vi "Autonomous Independent.vi"() -> ()   [LabVIEW 2016]
doc: "This VI is called when autonomous begins, and will automatically be terminated when autonomous ends. You can carry out timed or sensor driven robot movement independently without needing to return to the caller."
uses:
  2_8_17/Auto_Action.ctl
  <vilib>/Rock Robotics/WPI/Solenoid/WPI_SolenoidValue.ctl
  <vilib>/Rock Robotics/Network Tables/NT Read Number.vi
  <vilib>/Rock Robotics/WPI/Ultrasonic/WPI_SonarSRF04DigitalRefNum Registry Get.vi
  <vilib>/Rock Robotics/WPI/Ultrasonic/WPI_SonarSRF04DigitalGetRange.vi
  FRC SimulatedRSC/Positions.vi
panel:
  in  "Value":T1=enum."Forward"
  out "Auto Mode":dbl=3.0
  in  "Auton_Modes":T3(array[cluster])=[{"Actions"=[{"Effort"=0.55, "Duration"=3.5, "Action"=enum."Nothing"}, {"Effort"=0.0, "Duration"=0.0, "Action"=enum."Nothing"}]}, {"Actions"=[{"Effort"=0.0, "Duration"=1.0, "Action"=enum."Nothing"}, {"Effort"=0.75, "Duration"=5.0, "Action"=enum."Nothing"}, {"Effort"=0.0, "Duration"=1.0, "Action"=enum."Nothing"}]}, {"Actions"=[{"Effort"=1.0, "Duration"=3.0, "Action"=enum."Nothing"}, {"Effort"=0.0, "Duration"=1.0, "Action"=enum."Nothing"}, {"Effort"=0.75, "Duration"=3.5, "Action"=enum."Nothing"}, {"Effort"=0.0, "Duration"=1.0, "Action"=enum."Nothing"}]}, {"Actions"=[{"Effort"=0.0, "Duration"=0.5, "Action"=enum."Nothing"}, {"Effort"=0.8, "Duration"=5.28, "Action"=enum."Nothing"}, {"Effort"=0.0, "Duration"=1.0, "Action"=enum."Nothing"}, {"Effort"=-0.8, "Duration"=1.8, "Action"=enum."Nothing"}, {"Effort"=0.0, "Duration"=0.1, "Action"=enum."Nothing"}, {"Effort"=0.8, "Duration"=1.75, "Action"=enum."Nothing"}, {"Effort"=0.0, "Duration"=0.5, "Action"=enum."Nothing"}, {"Effort"=0.0, "Duration"=4.0, "Action"=enum."Nothing"}]}, {"Actions"=[{"Effort"=0.0, "Duration"=0.0, "Action"=enum."Nothing"}, {"Effort"=1.0, "Duration"=0.1, "Action"=enum."Nothing"}, {"Effort"=0.0, "Duration"=0.1, "Action"=enum."Nothing"}, {"Effort"=1.0, "Duration"=3.0, "Action"=enum."Nothing"}]}, {"Actions"=[{"Effort"=0.0, "Duration"=0.0, "Action"=enum."Nothing"}, {"Effort"=1.0, "Duration"=0.1, "Action"=enum."Nothing"}, {"Effort"=0.0, "Duration"=0.1, "Action"=enum."Nothing"}, {"Effort"=1.0, "Duration"=3.0, "Action"=enum."Nothing"}]}, {"Actions"=[{"Effort"=0.55, "Duration"=4.0, "Action"=enum."Nothing"}, {"Effort"=0.0, "Duration"=1.0, "Action"=enum."Nothing"}, {"Effort"=-0.5, "Duration"=0.6, "Action"=enum."Nothing"}, {"Effort"=0.75, "Duration"=1.0, "Action"=enum."Nothing"}, {"Effort"=0.0, "Duration"=1.0, "Action"=enum."Nothing"}, {"Effort"=0.75, "Duration"=3.0, "Action"=enum."Nothing"}]}, {"Actions"=[{"Effort"=0.0, "Duration"=0.5, "Action"=enum."Nothing"}, {"Effort"=0.55, "Duration"=4.25, "Action"=enum."Nothing"}, {"Effort"=0.0, "Duration"=0.0, "Action"=enum."Nothing"}, {"Effort"=0.0, "Duration"=0.3, "Action"=enum."Nothing"}, {"Effort"=0.9, "Duration"=2.0, "Action"=enum."Nothing"}]}, {"Actions"=[{"Effort"=0.0, "Duration"=0.0, "Action"=enum."Nothing"}]}]
  # "Nothing"
  # "Boiler Side Gear"
  # "Middle Gear"
  # "Farside Gear"
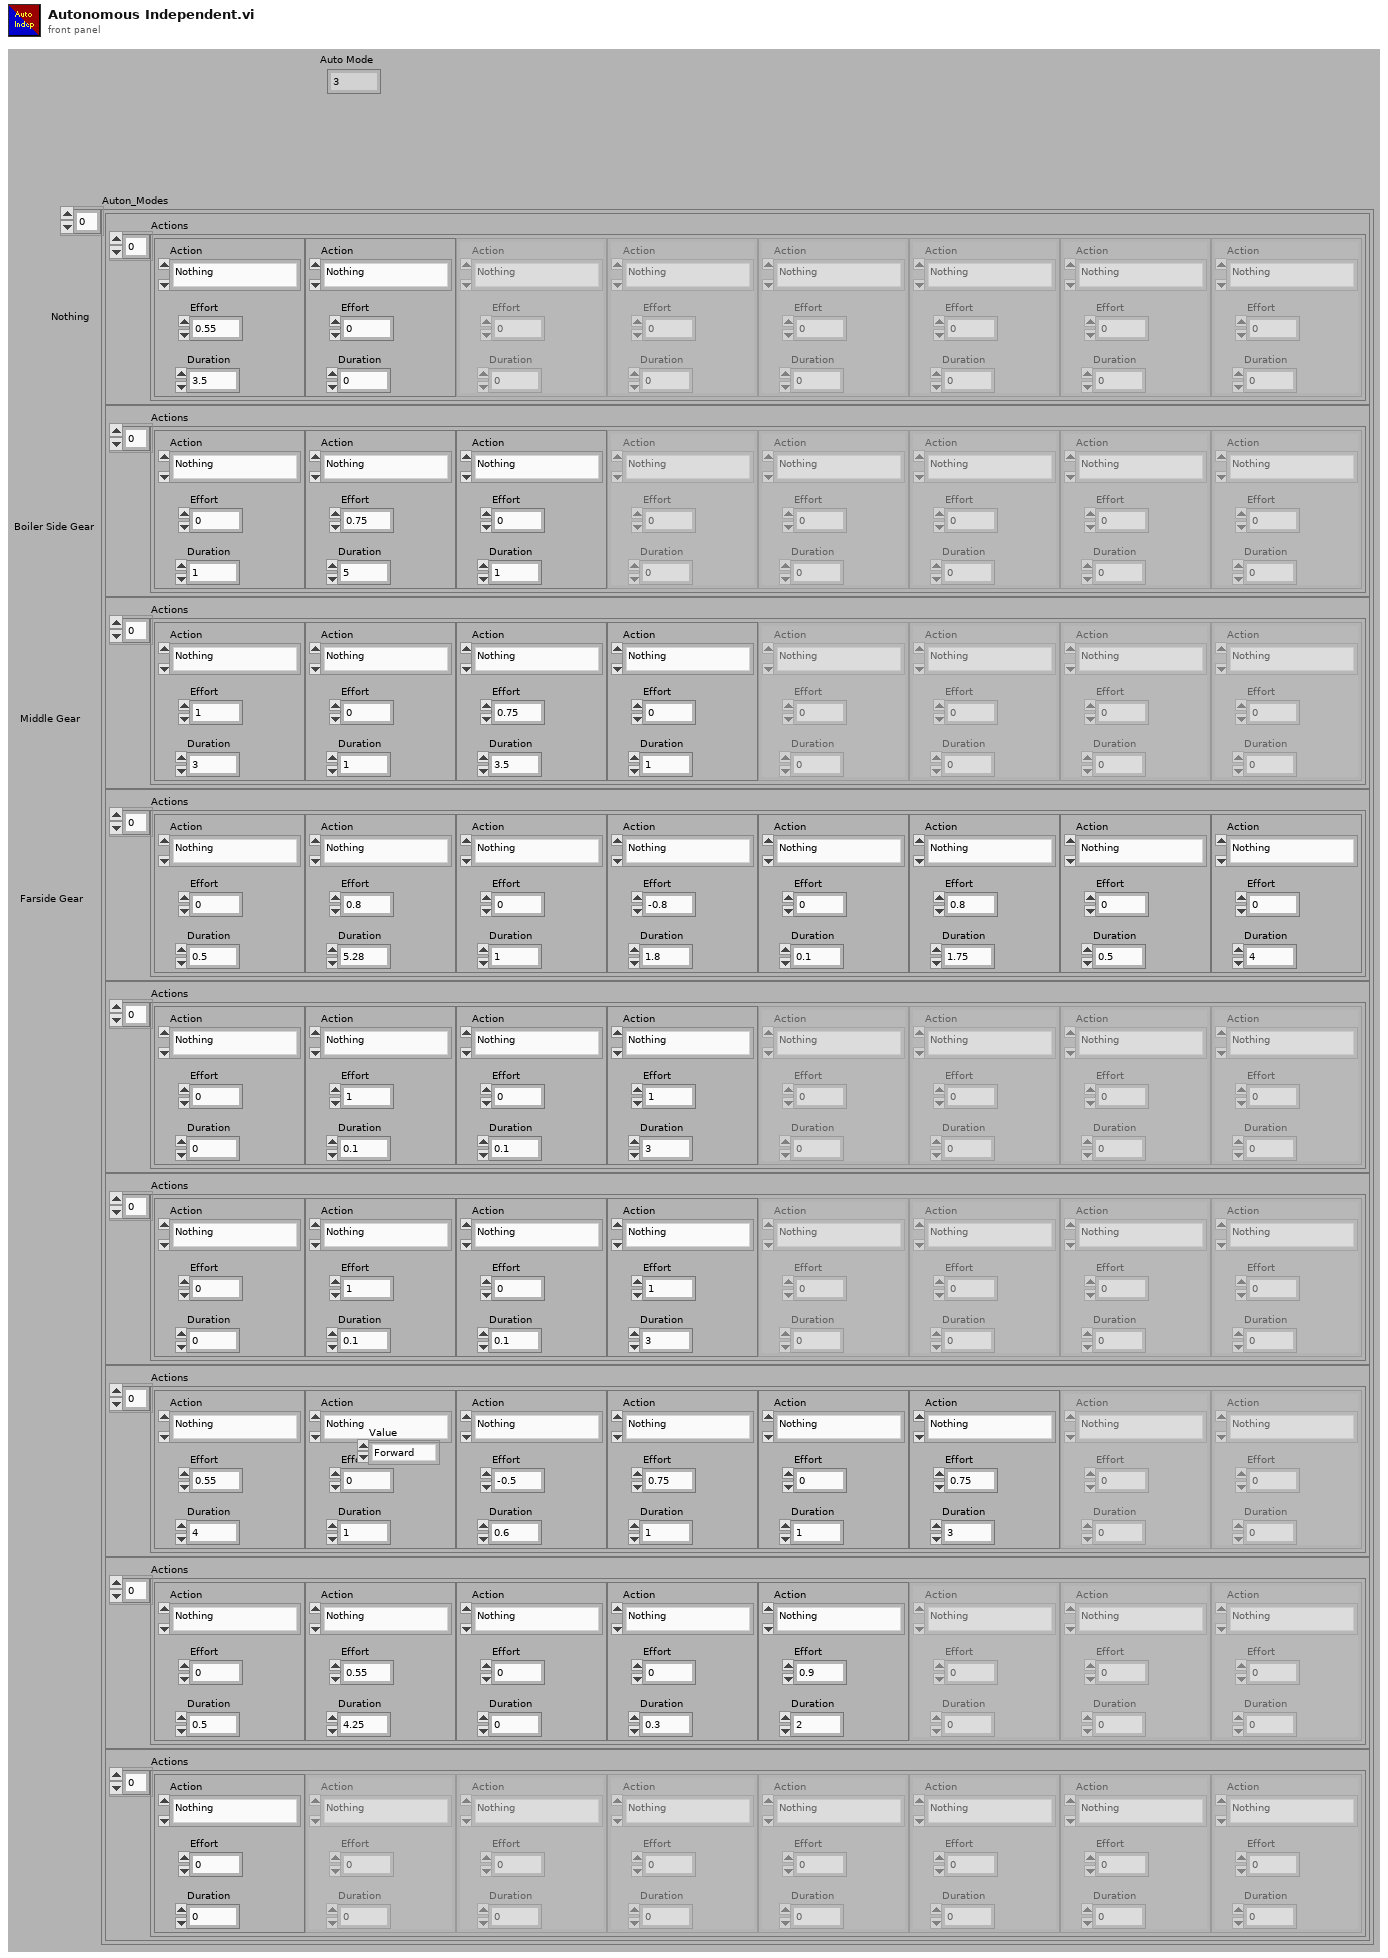
[diagram p1: front panel]
types:
  T1 = typedef "WPI_SolenoidValue.ctl" = enum16{"Off", "On", "Forward", "Reverse"}
  T2 = typedef "Auto_Action.ctl" = enum16{"Nothing", "Drive", "Vision Correction", "Turn", "Gear0", "Gear1", "Climb", "Intake", "Index", "Shoot", "Test", "Drive Encoder Reset", "Gyro Reset"}
  T3 = cluster{"Actions":cluster{"Effort":dbl, "Duration":dbl, "Action":T2}[]}[]
  T4 = cluster{"Actions":cluster{"Effort":dbl, "Duration":dbl, "Action":T2}[]}
  T5 = cluster{"Effort":dbl, "Duration":dbl, "Action":T2}[]
  T6 = typedef "WPI_MotorControlDeviceRef.ctl" = cluster{"DeviceStatus":errorcluster, "Type":T7, "PWM":cluster{"PWM Channel":T8, "DeadBand":T9}, "CAN":cluster{"Device Number":u8, "SetOutput VI Ref":variant, "GetOutput VI Ref":variant, "Enable VI Ref":variant, "Disable VI Ref":variant, "Data":variant}, "Invert":bool}
  T7 = typedef "WPI_MotorControlType.ctl" = enum16{"PWM", "CAN"}
  T8 = typedef "FPGA_DIOPWMChannel.ctl" = enum8{"PWM 0", "PWM 1", "PWM 2", "PWM 3", "PWM 4", "PWM 5", "PWM 6", "PWM 7", "PWM 8", "PWM 9", "PWM MXP 0", "PWM MXP 1", "PWM MXP 2", "PWM MXP 3", "PWM MXP 4", "PWM MXP 5", "PWM MXP 6", "PWM MXP 7", "PWM MXP 8", "PWM MXP 9", "Invalid"}
  T9 = typedef "WPI_PWMDeadband.ctl" = cluster{"Name":string, "maxPositivePwm":i32, "minPositivePwm":i32, "centerPwm":i32, "maxNegativePwm":i32, "minNegativePwm":i32, "angularRange":u16}
  T10 = typedef "WPI_UltrasonicDeviceRef.ctl" = cluster{"DevStatus":errorcluster, "Ping Channel":T11, "Echo Channel":T11, "CntIndex":T12}
  T11 = typedef "FPGA_DIOChannel.ctl" = enum8{"DIO 0", "DIO 1", "DIO 2", "DIO 3", "DIO 4", "DIO 5", "DIO 6", "DIO 7", "DIO 8", "DIO 9", "DIO MXP 0", "DIO MXP 1", "DIO MXP 2", "DIO MXP 3", "DIO MXP 4", "DIO MXP 5", "DIO MXP 6", "DIO MXP 7", "DIO MXP 8", "DIO MXP 9", "DIO MXP 10", "DIO MXP 11", "DIO MXP 12", "DIO MXP 13", "DIO MXP 14", "DIO MXP 15", "SPI Port CS1", "SPI Port CS2", "SPI Port CS3", "SPI Port MISO", "SPI Port MOSI", "Invalid"}
  T12 = typedef "FPGA_CounterCtrSystemIndex.ctl" = enum8{"Ctr 0", "Ctr 1", "Ctr 2", "Ctr 3", "Ctr 4", "Ctr 5", "Ctr 6", "Ctr 7", "Invalid"}
  T13 = typedef "WPI_GyroDevRef.ctl" = cluster{"DevStatus":errorcluster, "Analog Channel":T14, "Offset":dbl, "Gain (VoltsPerDegree/Second)":dbl, "Gyro Type":enum16{"Analog", "XRS450"}, "Handle":i32, "SPI Bus":T15, "Device Found":bool, "Sample Rate":dbl, "Calibrate On Open":bool}
  T14 = typedef "FPGA_AIChannel.ctl" = enum8{"AI 0", "AI 1", "AI 2", "AI 3", "AI MXP 0", "AI MXP 1", "AI MXP 2", "AI MXP 3", "Invalid"}
  T15 = typedef "spi_bus.ctl" = enum16{"SPI On-Board, CS0", "SPI On-Board, CS1", "SPI On-Board, CS2", "SPI On-Board, CS3", "SPI MXP", "Invalid"}
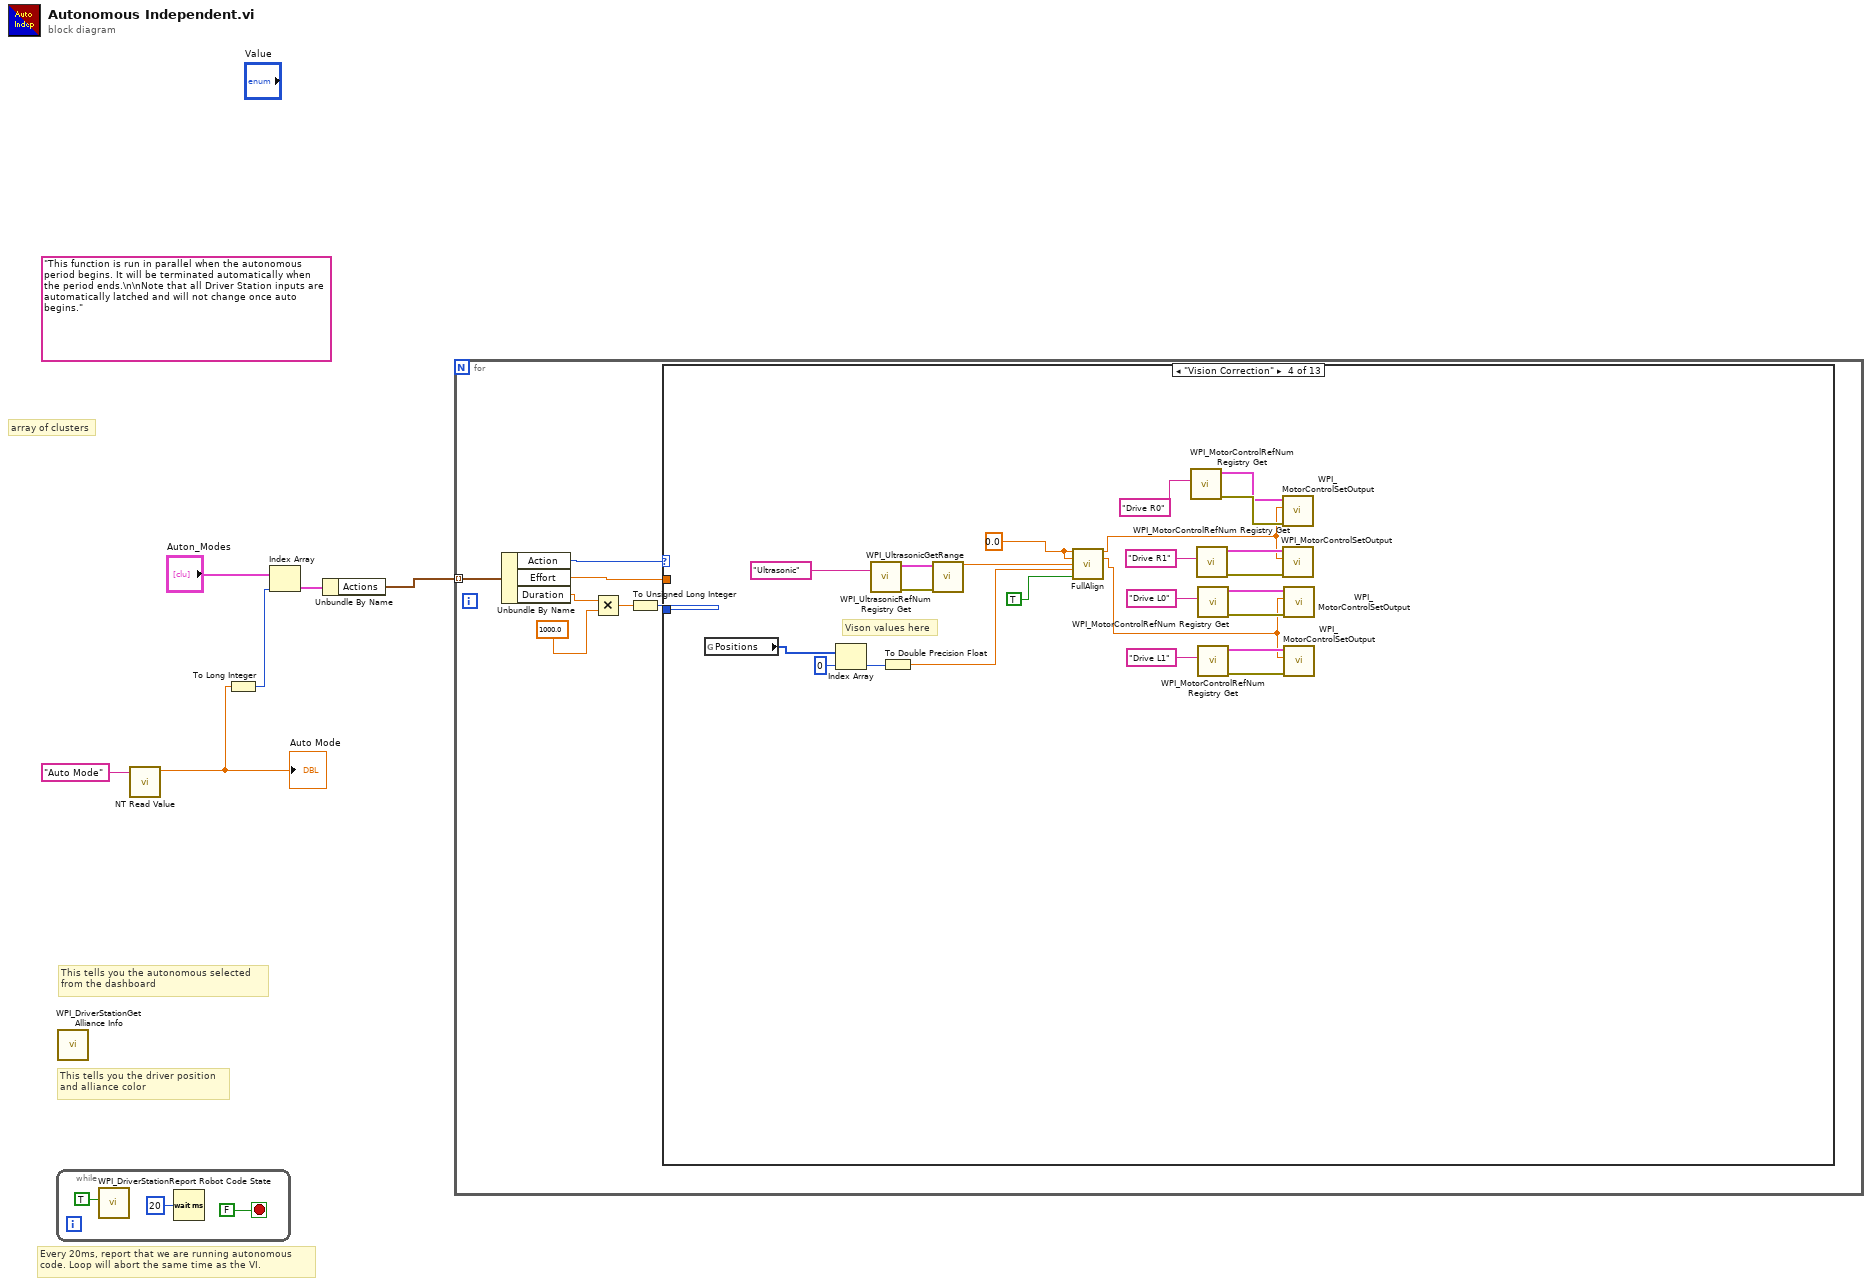
[diagram p0: block diagram]
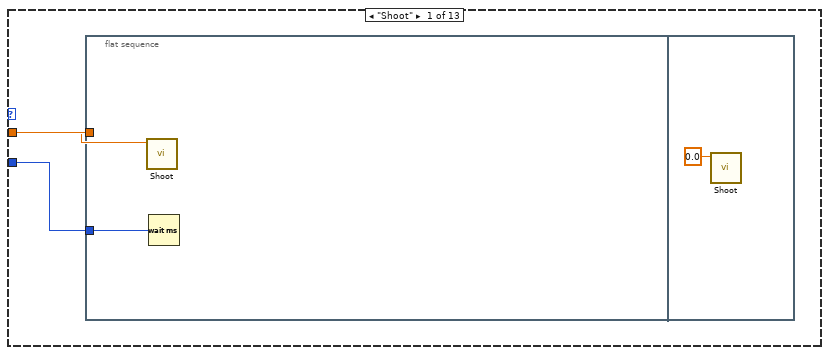
[diagram p2: hidden frame]
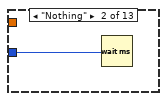
[diagram p3: hidden frame]
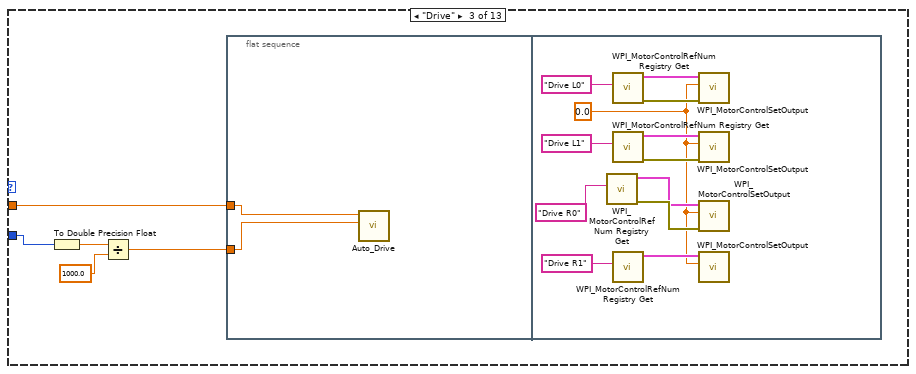
[diagram p4: hidden frame]
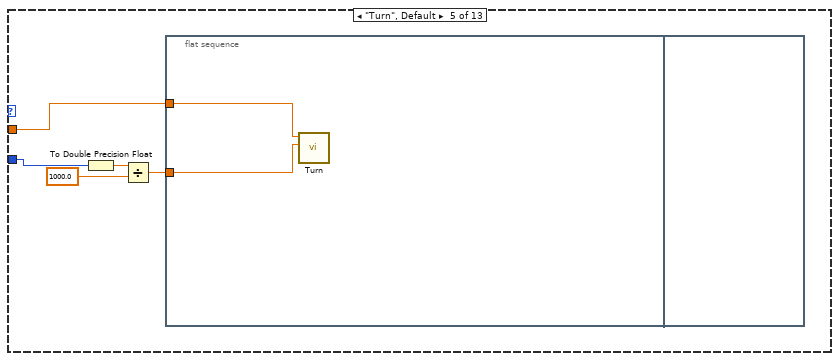
[diagram p5: hidden frame]
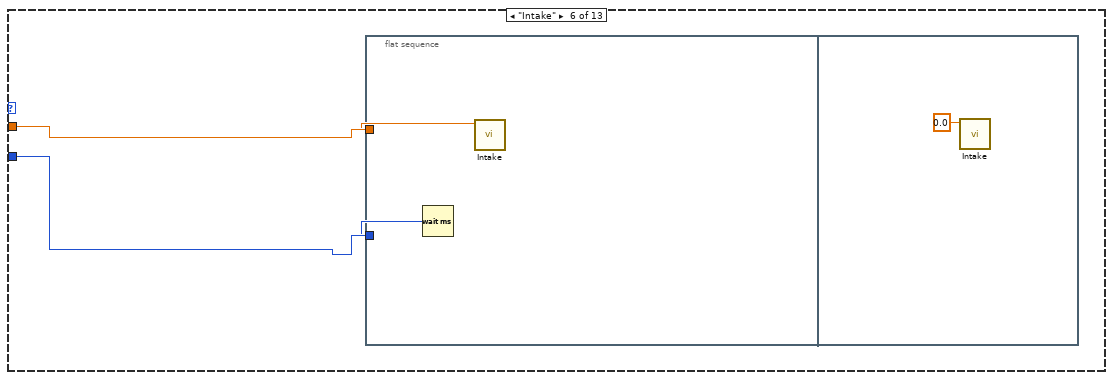
[diagram p6: hidden frame]
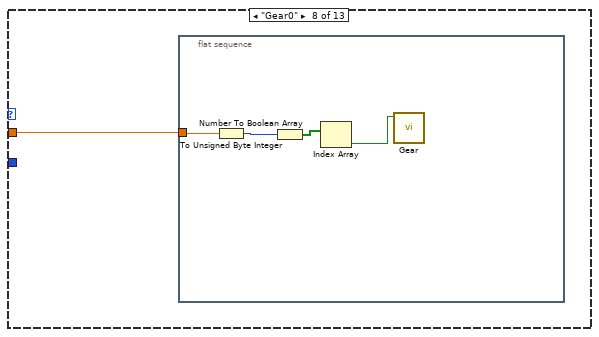
[diagram p8: hidden frame]
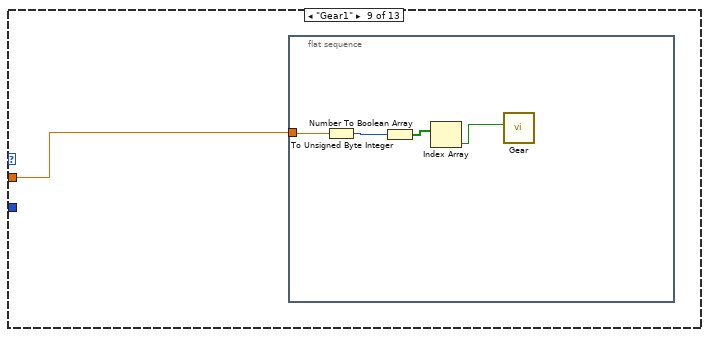
[diagram p9: hidden frame]
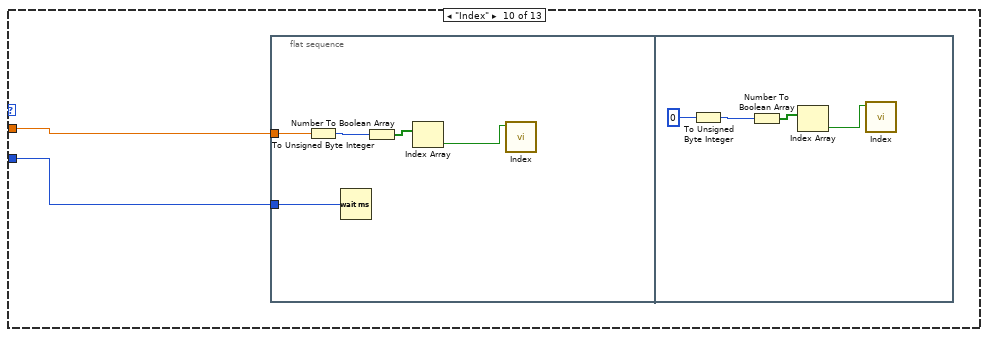
[diagram p10: hidden frame]
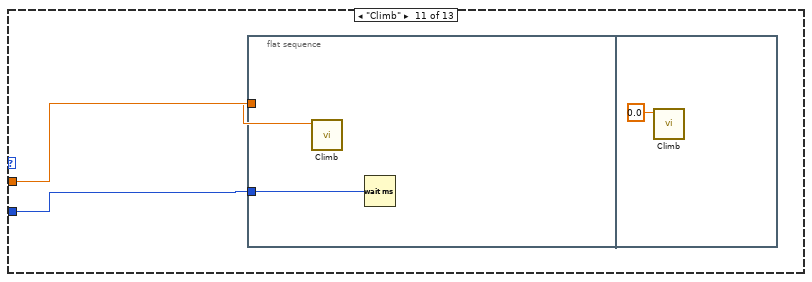
[diagram p11: hidden frame]
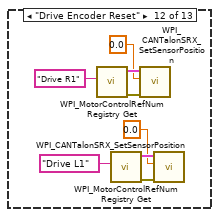
[diagram p12: hidden frame]
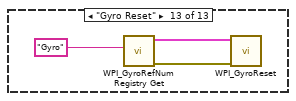
[diagram p13: hidden frame]
diagram:
  (unwired) "This function is run in parallel when the autonomous period begins. It will be terminated automatically when the period ends.\n\nNote that all Driver Station inputs are automatically latched and will not change once auto begins."
  # "This tells you the autonomous selected\nfrom the dashboard"
  # "array of clusters"
  # "Every 20ms, report that we are running autonomous\ncode. Loop will abort the same time as the VI."
  # "This tells you the driver position\nand alliance color"
  n1 = while {
    stop <- FALSE stop-if-true
    n2 = call <vilib>:"WPI_DriverStationReport Robot Code State.vi"("Autonomous"=TRUE) -> ()  [unwired: 10 in, 1 out]
    n3 = Wait (ms)(milliseconds to wait=u32 20) -> ()  [unwired: 1 out]
  }
  n4 = call <vilib>:"WPI_DriverStationGet Alliance Info.vi"() -> ()  [unwired: 12 out]
  n5 = call-poly <vilib>:"NT Read Value.vi"("Name"="Auto Mode") -> ("Numeric"=w1:dbl)  [unwired: 9 in, 1 out]
  "Auto Mode" <- w1
  n6 = To Long Integer(number=w1) -> (32bit integer=w3:i32)
  n7 = Index Array(array="Auton_Modes", index=w3) -> (element=w5:T4)
  n8 = Unbundle By Name(w5) -> ("Actions"=w6:T5)
  n9 = for {
    tunnel: w6 -> [w16] mode=indexing
    n10 = Unbundle By Name(w16) -> ("Action"=w15:T2, "Effort"=w14:dbl, "Duration"=w13:dbl)
    n11 = Multiply(x=w13, y=1000.0) -> (x*y=w11:dbl)
    n12 = To Unsigned Long Integer(number=w11) -> (unsigned 32bit integer=w10:u32)
    n13 = case shown="\"Vision Correction\"" w15 {
      tunnel: w14 -> [w18 _ w27 _ w70 w74 _ w78 w83 w88 w100 _ _]
      tunnel: w10 -> [w17 w22 w26 _ w69 w73 _ _ _ w89 w99 _ _]
      frame "Shoot" {
        n14 = flat-sequence {
          tunnel: w18 -> [w20]
          tunnel: w17 -> [w19]
          frame #0 {
            n15 = call "Shoot.vi"("Set RPM"=w20) -> ()  [unwired: 11 in]
            n16 = Wait (ms)(milliseconds to wait=w19) -> ()  [unwired: 1 out]
          }
          frame #1 {
            n17 = call "Shoot.vi"("Set RPM"=0.0 ("Effort")) -> ()  [unwired: 11 in]
          }
        }
      }
      frame "Nothing" {
        n18 = Wait (ms)(milliseconds to wait=w22) -> ()  [unwired: 1 out]
      }
      frame "Drive" {
        n19 = To Double Precision Float(number=w26) -> (double precision float=w25:dbl)
        n20 = Divide(x=w25, y=1000.0) -> (x/y=w23:dbl)
        n21 = flat-sequence {
          tunnel: w27 -> [w29]
          tunnel: w23 -> [w28]
          frame #0 {
            n22 = call "Auto_Drive.vi"("Duration"=w28, "Drive Effort"=w29) -> ()  [unwired: 10 in]
          }
          frame #1 {
            w30 = 0.0 ("Drive L")
            n23 = call <vilib>:"WPI_MotorControlRefNum Registry Get.vi"("refnum name"="Drive R0") -> ("error out"=w35:errorcluster, "MotorControlDevRef"=w31:T6)  [unwired: 9 in]
            n24 = call <vilib>:"WPI_MotorControlRefNum Registry Get.vi"("refnum name"="Drive L0") -> ("error out"=w36:errorcluster, "MotorControlDevRef"=w37:T6)  [unwired: 9 in]
            n25 = call <vilib>:"WPI_MotorControlRefNum Registry Get.vi"("refnum name"="Drive L1") -> ("error out"=w40:errorcluster, "MotorControlDevRef"=w39:T6)  [unwired: 9 in]
            n26 = call <vilib>:"WPI_MotorControlRefNum Registry Get.vi"("refnum name"="Drive R1") -> ("MotorControlDevRef"=w33:T6)  [unwired: 9 in, 1 out]
            n27 = call <vilib>:"WPI_MotorControlSetOutput.vi"("error in (no error)"=w36, "Output"=w30, "MotorControlDevRef"=w37) -> ()  [unwired: 6 in, 3 out]
            n28 = call <vilib>:"WPI_MotorControlSetOutput.vi"("error in (no error)"=w40, "Output"=w30, "MotorControlDevRef"=w39) -> ()  [unwired: 6 in, 3 out]
            n29 = call <vilib>:"WPI_MotorControlSetOutput.vi"("error in (no error)"=w35, "Output"=w30, "MotorControlDevRef"=w31) -> ()  [unwired: 6 in, 3 out]
            n30 = call <vilib>:"WPI_MotorControlSetOutput.vi"("Output"=w30, "MotorControlDevRef"=w33) -> ()  [unwired: 7 in, 3 out]
          }
        }
      }
      frame "Vision Correction" {
        w45 = 0.0
        # "Vison values here"
        n31 = global read "Positions.vi" "Positions"() -> (w48:i32[])
        n32 = Index Array(array=w48, index=0) -> (element=w49:i32)
        n33 = call-poly <vilib>:"WPI_UltrasonicRefNum Registry Get.vi"("refnum name"="Ultrasonic") -> ("error out"=w65:errorcluster, "SonarSRF04DevRef"=w64:T10)  [unwired: 9 in]
        n34 = To Double Precision Float(number=w49) -> (double precision float=w44:dbl)
        n35 = call-poly <vilib>:"WPI_UltrasonicGetRange.vi"("error in (no error)"=w65, "SonarSRF04DevRef"=w64) -> ("Distance"=w43:dbl)  [unwired: 7 in, 2 out]
        n36 = call "FullAlign.vi"("Joystick 0"=w45, "Joystick 1"=w45, "Distance"=w43, "Angle"=w44, "Button"=TRUE) -> ("Right Motor"=w47:dbl, "Left Motor"=w46:dbl)  [unwired: 8 in, 1 out]
        n37 = call <vilib>:"WPI_MotorControlRefNum Registry Get.vi"("refnum name"="Drive R0") -> ("error out"=w57:errorcluster, "MotorControlDevRef"=w53:T6)  [unwired: 9 in]
        n38 = call <vilib>:"WPI_MotorControlRefNum Registry Get.vi"("refnum name"="Drive R1") -> ("error out"=w52:errorcluster, "MotorControlDevRef"=w55:T6)  [unwired: 9 in]
        n39 = call <vilib>:"WPI_MotorControlRefNum Registry Get.vi"("refnum name"="Drive L0") -> ("error out"=w58:errorcluster, "MotorControlDevRef"=w59:T6)  [unwired: 9 in]
        n40 = call <vilib>:"WPI_MotorControlRefNum Registry Get.vi"("refnum name"="Drive L1") -> ("error out"=w62:errorcluster, "MotorControlDevRef"=w61:T6)  [unwired: 9 in]
        n41 = call <vilib>:"WPI_MotorControlSetOutput.vi"("error in (no error)"=w57, "Output"=w47, "MotorControlDevRef"=w53) -> ()  [unwired: 6 in, 3 out]
        n42 = call <vilib>:"WPI_MotorControlSetOutput.vi"("error in (no error)"=w52, "Output"=w47, "MotorControlDevRef"=w55) -> ()  [unwired: 6 in, 3 out]
        n43 = call <vilib>:"WPI_MotorControlSetOutput.vi"("error in (no error)"=w58, "Output"=w46, "MotorControlDevRef"=w59) -> ()  [unwired: 6 in, 3 out]
        n44 = call <vilib>:"WPI_MotorControlSetOutput.vi"("error in (no error)"=w62, "Output"=w46, "MotorControlDevRef"=w61) -> ()  [unwired: 6 in, 3 out]
      }
      frame "Turn", Default {
        n45 = To Double Precision Float(number=w69) -> (double precision float=w68:dbl)
        n46 = Divide(x=w68, y=1000.0) -> (x/y=w66:dbl)
        n47 = flat-sequence {
          tunnel: w70 -> [w72]
          tunnel: w66 -> [w71]
          frame #0 {
            n48 = call "Turn.vi"("Angle"=w71, "Effort"=w72) -> ()  [unwired: 10 in]
          }
          frame #1 {
          }
        }
      }
      frame "Intake" {
        n49 = flat-sequence {
          tunnel: w74 -> [w76]
          tunnel: w73 -> [w75]
          frame #0 {
            n50 = Wait (ms)(milliseconds to wait=w75) -> ()  [unwired: 1 out]
            n51 = call "Intake.vi"("Effort"=w76) -> ()  [unwired: 11 in]
          }
          frame #1 {
            n52 = call "Intake.vi"("Effort"=0.0) -> ()  [unwired: 11 in]
          }
        }
      }
      frame "Test" {
      }
      frame "Gear0" {
        n53 = flat-sequence {
          tunnel: w78 -> [w82]
          frame #0 {
            n54 = To Unsigned Byte Integer(number=w82) -> (unsigned 8bit integer=w81:u8)
            n55 = Number To Boolean Array(number=w81) -> (Boolean array=w80:bool[])
            n56 = Index Array(array=w80) -> (element=w79:bool)  [unwired: 1 in]
            n57 = call "Gear.vi"("Gear0?"=w79) -> ()  [unwired: 11 in]
          }
        }
      }
      frame "Gear1" {
        n58 = flat-sequence {
          tunnel: w83 -> [w87]
          frame #0 {
            n59 = To Unsigned Byte Integer(number=w87) -> (unsigned 8bit integer=w86:u8)
            n60 = Number To Boolean Array(number=w86) -> (Boolean array=w85:bool[])
            n61 = Index Array(array=w85) -> (element=w84:bool)  [unwired: 1 in]
            n62 = call "Gear.vi"("Gear1?"=w84) -> ()  [unwired: 11 in]
          }
        }
      }
      frame "Index" {
        n63 = flat-sequence {
          tunnel: w89 -> [w91]
          tunnel: w88 -> [w90]
          frame #0 {
            n64 = To Unsigned Byte Integer(number=w90) -> (unsigned 8bit integer=w94:u8)
            n65 = Wait (ms)(milliseconds to wait=w91) -> ()  [unwired: 1 out]
            n66 = Number To Boolean Array(number=w94) -> (Boolean array=w93:bool[])
            n67 = Index Array(array=w93) -> (element=w92:bool)  [unwired: 1 in]
            n68 = call "Index.vi"("Index?"=w92) -> ()  [unwired: 11 in]
          }
          frame #1 {
            n69 = To Unsigned Byte Integer(number=u8 0) -> (unsigned 8bit integer=w97:u8)
            n70 = Number To Boolean Array(number=w97) -> (Boolean array=w98:bool[])
            n71 = Index Array(array=w98) -> (element=w95:bool)  [unwired: 1 in]
            n72 = call "Index.vi"("Index?"=w95) -> ()  [unwired: 11 in]
          }
        }
      }
      frame "Climb" {
        n73 = flat-sequence {
          tunnel: w100 -> [w102]
          tunnel: w99 -> [w101]
          frame #0 {
            n74 = call "Climb.vi"("Effort"=w102) -> ()  [unwired: 11 in]
            n75 = Wait (ms)(milliseconds to wait=w101) -> ()  [unwired: 1 out]
          }
          frame #1 {
            n76 = call "Climb.vi"("Effort"=0.0) -> ()  [unwired: 11 in]
          }
        }
      }
      frame "Drive Encoder Reset" {
        n77 = call <vilib>:"WPI_MotorControlRefNum Registry Get.vi"("refnum name"="Drive R1") -> ("error out"=w106:errorcluster, "MotorControlDevRef"=w105:T6)  [unwired: 9 in]
        n78 = call <vilib>:"WPI_MotorControlRefNum Registry Get.vi"("refnum name"="Drive L1") -> ("error out"=w108:errorcluster, "MotorControlDevRef"=w109:T6)  [unwired: 9 in]
        n79 = call <vilib>:"WPI_CANTalonSRX_SetSensorPosition.vi"("error in (no error)"=w106, "New Sensor Position"=0.0, "CAN Talon SRX Ref"=w105) -> ()  [unwired: 7 in, 2 out]
        n80 = call <vilib>:"WPI_CANTalonSRX_SetSensorPosition.vi"("error in (no error)"=w108, "New Sensor Position"=0.0, "CAN Talon SRX Ref"=w109) -> ()  [unwired: 7 in, 2 out]
      }
      frame "Gyro Reset" {
        n81 = call <vilib>:"WPI_GyroRefNum Registry Get.vi"("refnum name"="Gyro") -> ("error out"=w113:errorcluster, "GyroDevRef"=w114:T13)  [unwired: 9 in]
        n82 = call <vilib>:"WPI_GyroReset.vi"("error in"=w113, "GyroDevRef"=w114) -> ()  [unwired: 8 in, 2 out]
      }
    }
  }
